vi "Teststand Post Sub Steps STP Sent Command.vi"(9 "Socket No":u16=1, 10 "STP Set Profile Data in":T1={"ECU CAN Port"="CAN1", "CMD"=133, "CAN Write Data"=[], "+veResponseCode"=160} {"+veResponseCode" format="%.0x"; "CMD" items=["TSW_VERSION(130)"=130, "WAIT_EVENT(132)"=132, "SEQUENCER(133)"=133, "TSW_RESET(150)"=150, "CONFIG_ECU(151)"=151, "TEST_CORE (152)"=152, "TEST_WATCHDOG (153)"=153, "TEST_MONITORING (154)"=154, "READ_MEMORY (162)"=162, "WRITE_ERASE_MEMORY (164)"=164, "COMM_EXTERNAL (190)"=190, "COMM_INTERNAL (195)"=195, "GET_ANALOG_INPUT (210)"=210, "GET_DIGITAL_INPUT (211)"=211, "GET_FREQUENCY_INPUT (212)"=212, "TEST_INPUT_STRUCTURE (214)"=214, "GENERATE_OUTPUT_SIGNAL (220)"=220, "GENERATE_SYNCHRONIZED_OUTPUT_SIGNALS (221)"=221, "eDCU_Specific (250)"=250]; "CAN Write Data" format="%.0x"}, 11 "Sequence Context In":refnum<k7>) -> (0 "error out":errorcluster, 1 "STP Error":T3, 2 "STP Data Out":T4, 3 "Report Text":string, 5 "PositiveResponse?":bool)   [LabVIEW 2023, in "LTT_TeststandSteptypes.lvlib"]
uses:
  LTT_TeststandSteptypes.lvlib
  Control/STP Out Data.ctl
  HardwareAbstractionLayer_LVOOP/CAN/CAN Application Protocols/STP Protocol_class/Ctrls/STP Error Cluster.ctl
  Control/STP Sent Command.ctl
  HardwareAbstractionLayer_LVOOP/CAN/CAN Application Protocols/STP Protocol_class/Ctrls/STP CMD.ctl
  HardwareAbstractionLayer_LVOOP/CAN/CAN Application Protocols/STP Protocol_class/Ctrls/STP Input Data.ctl
  HardwareAbstractionLayer_LVOOP/CAN/CAN Application Protocols/STP Protocol_class/STP Protocol.lvclass
panel:
  out "RequestTimeout?":bool
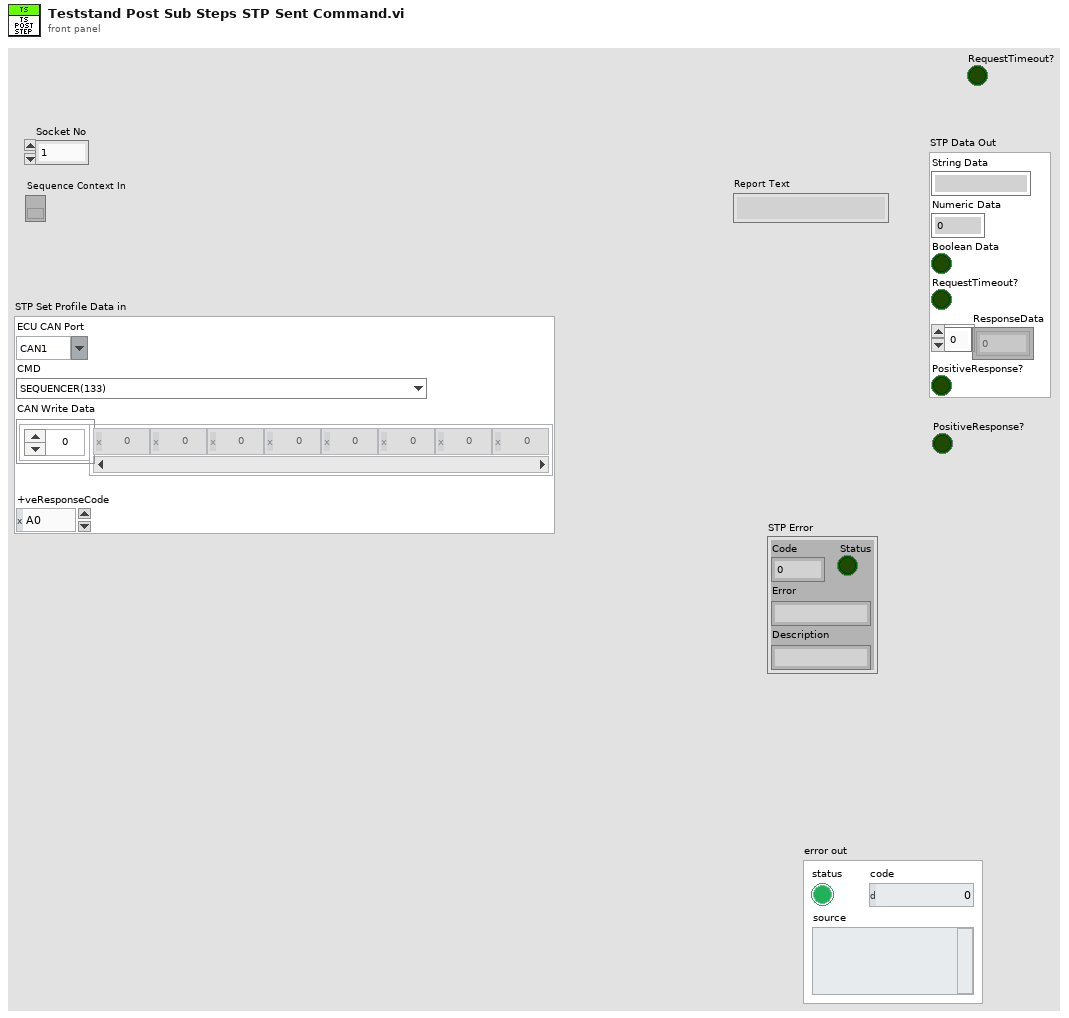
[diagram p1: front panel]
types:
  T1 = typedef "LTT_TeststandSteptypes.lvlib/STP Sent Command.ctl" = cluster{"ECU CAN Port":string, "CMD":T2, "CAN Write Data":u8[], "+veResponseCode":u8}
  T2 = typedef "HardwareAbstractionLayer_LVOOP.lvlib/CAN Application Protocols Lib.lvlib/STP Protocol.lvclass/STP CMD.ctl" = u8
  T3 = typedef "HardwareAbstractionLayer_LVOOP.lvlib/CAN Application Protocols Lib.lvlib/STP Protocol.lvclass/STP Error Cluster.ctl" = cluster{"Status":bool, "Code":u8, "Error":string, "Description":string}
  T4 = typedef "LTT_TeststandSteptypes.lvlib/STP Out Data.ctl" = cluster{"String Data":string, "Numeric Data":dbl, "Boolean Data":bool, "RequestTimeout?":bool, "ResponseData":u8[], "PositiveResponse?":bool}
  T5 = typedef "HardwareAbstractionLayer_LVOOP.lvlib/CAN Application Protocols Lib.lvlib/STP Protocol.lvclass/STP Input Data.ctl" = cluster{"TxID":u32, "RxID":u32, "CMD":T2, "RQ Data":u8[], "+veResponseCode":u8, "ResponseTimeout (S)":dbl}
  T6 = typedef "HardwareAbstractionLayer_LVOOP.lvlib/CAN HAL Lib.lvlib/CAN.lvclass/CAN Init Ctrl.ctl" = cluster{"XNET Interface":refnum<k21>, "Baud Rate":u64, "CAN:Termination":u32, "Echo Transmit?":bool, "scope (normal)":T7}
  T7 = typedef "XNET Control Scope.ctl" = u32
  T8 = cluster{"Refnum out":refnum<k21>, "CAN Init Data":T6, "CAN_RxID":u32, "CAN_TxID":u32, "Timeout":dbl}
  T9 = typedef "HardwareAbstractionLayer_LVOOP.lvlib/CAN Application Protocols Lib.lvlib/STP Protocol.lvclass/STP Output Data.ctl" = cluster{"ResponseData":u8[], "ResponseData(ASCII)":string, "PositiveResponse?":bool, "STP Error":T3}
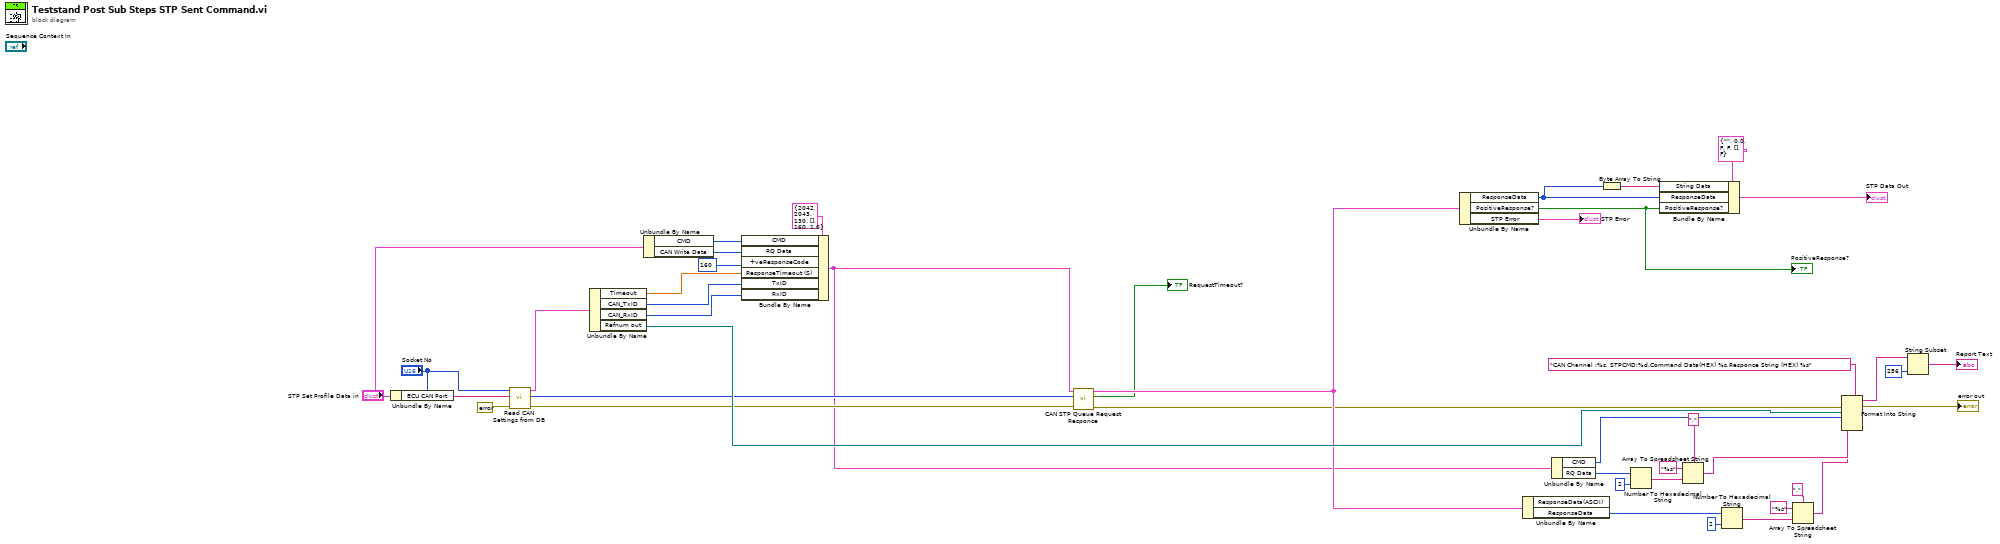
[diagram p0: block diagram]
diagram:
  n1 = Unbundle By Name("STP Set Profile Data in") -> ("ECU CAN Port"=w13:string)
  n2 = call "Read CAN Settings from DB.vi"("error in"=errorcluster {"status"=FALSE, "code"=0, "source"=""}, "ECU CAN Port"=w13, "Socket No"="Socket No") -> ("error out"=w5:errorcluster, "Read CAN Setting"=w11:T8)  [unwired: 7 in]
  n3 = Unbundle By Name(w11) -> ("Timeout"=w10:dbl, "CAN_TxID"=w9:u32, "CAN_RxID"=w8:u32, "Refnum out"=w7:refnum<k21>)
  n4 = Unbundle By Name("STP Set Profile Data in") -> ("CMD"=w41:T2, "CAN Write Data"=w40:u8[])
  n5 = Bundle By Name(cluster=T5 {"TxID"=2042, "RxID"=2043, "CMD"=130, "RQ Data"=[], "+veResponseCode"=160, "ResponseTimeout (S)"=1.0} ("STP Input Data"), "CMD"=w41, "RQ Data"=w40, "+veResponseCode"=u8 160, "ResponseTimeout (S)"=w10, "TxID"=w9, "RxID"=w8) -> (w2:T5)
  n6 = call "CAN STP Queue Request Responce.vi"("error in (no error)"=w5, "Socket No"="Socket No", "STP Input Data"=w2) -> ("error out"=w4:errorcluster, "RequestTimeout?"=→"RequestTimeout?":bool, "STP Output Data"=w6:T9)  [unwired: 6 in]
  n7 = Unbundle By Name(w6) -> ("ResponseData"=w36:u8[], "PositiveResponse?"=w33:bool, "STP Error"=→"STP Error":T3)
  "PositiveResponse?" <- w33
  n8 = Unbundle By Name(w6) -> ("ResponseData"=w20:u8[])  [unwired: 1 out]
  n9 = Unbundle By Name(w2) -> ("CMD"=w30:T2, "RQ Data"=w22:u8[])
  n10 = Byte Array To String(unsigned byte array=w36) -> (string=w37:string)
  n11 = Number To Hexadecimal String(1:i16 2 ("width (-)"), 2:w22) -> (0:w26:string[])
  n12 = Bundle By Name(cluster=T4 {"String Data"="", "Numeric Data"=0.0, "Boolean Data"=FALSE, "RequestTimeout?"=FALSE, "ResponseData"=[], "PositiveResponse?"=FALSE} ("STP Data Out"), "String Data"=w37, "ResponseData"=w36, "PositiveResponse?"=w33) -> (→"STP Data Out":T4)
  n13 = Array To Spreadsheet String(delimiter (Tab)=",", array=w26, 3:"%s" ("format string")) -> (spreadsheet string=w28:string)
  n14 = Number To Hexadecimal String(1:i16 2 ("width (-)"), 2:w20) -> (0:w19:string[])
  n15 = Array To Spreadsheet String(delimiter (Tab)=",", array=w19, 3:"%s" ("format string")) -> (spreadsheet string=w18:string)
  n16 = Format Into String(format string="CAN Channel :%s, STPCMD:%d,Command Data(HEX) %s,Responce String (HEX) %s", error in=w4, w7, w30, w28, w18) -> (resulting string=w17:string, error out=→"error out":errorcluster)  [unwired: 1 in]
  n17 = String Subset(string=w17, length (rest)=256 ("length (rest)")) -> (substring=→"Report Text":string)  [unwired: 1 in]
